vi "Drive_Loop_Drive_Distance.vi"(6 "Distance":dbl, 8 "Absolute Angle? 4":bool, 9 "Angle 3":dbl, 10 "Power 3":dbl, 11 "Drive Loop Cluster":T1) -> ()   [LabVIEW 2016]
doc: "Help file writen by FRC Team 836 - The RoboBees\n\nThis VI commands the robot to drive a certain distance.\n\nThis VI writes the \"Drive Distance\" command, power level #3, Distance to travel, and if it is an absoulute angle to the\nDrive Command RT FIFO in Drive Loop Cluster.\n\nThe RT FIFO has to be initialized using the \"Drive_Loop_Initialize_w_Help\" VI"
uses:
  <userlib>/836-libraries/Drive/Drive_Code/Drive_Code_Support/Drive_Code_Bundle.ctl
  <userlib>/836-libraries/Drive/Drive_Code/Drive_Code_Support/Sensor_Cluster.ctl
  <userlib>/836-libraries/Drive/Drive_Code/Drive_Code_Support/Camera_Cluster.ctl
  <userlib>/836-libraries/Drive/Drive_Code/Drive_Code_Support/Drive_Code_Notifier.ctl
  <userlib>/836-libraries/Drive/Drive_Code/Drive_Code_Support/Drive_Code_Command.ctl
  <userlib>/836-libraries/Drive/Drive_Code/Logging_Data.ctl
  <userlib>/836-libraries/Drive/Drive_Code/Drive_Code_Support/Drive_Code_PID_Bundle.ctl
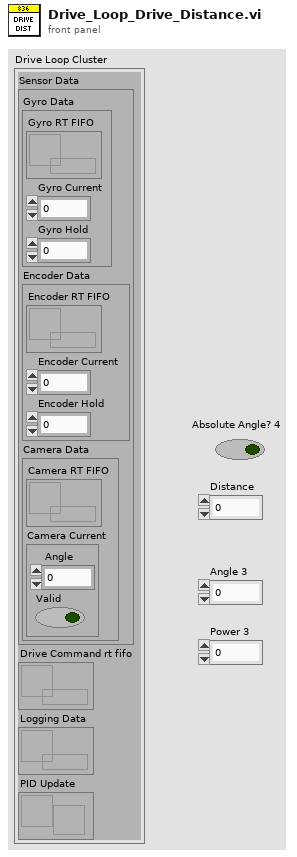
[diagram p1: front panel]
types:
  T1 = typedef "Drive_Code_Bundle.ctl" = cluster{"Sensor Data":T2, "Drive Command rt fifo":refnum<k33>, "Logging Data":refnum<k33>, "PID Update":refnum<notifier>}
  T2 = typedef "Sensor_Cluster.ctl" = cluster{"Gyro Data":cluster{"Gyro RT FIFO":refnum<k33>, "Gyro Current":dbl, "Gyro Hold":dbl}, "Encoder Data":cluster{"Encoder RT FIFO":refnum<k33>, "Encoder Current":dbl, "Encoder Hold":dbl}, "Camera Data":cluster{"Camera RT FIFO":refnum<k33>, "Camera Current":T3}}
  T3 = typedef "Camera_Cluster.ctl" = cluster{" Angle":dbl, "Valid":bool}
  T4 = typedef "Drive_Code_Command.ctl" = enum16{"Do Nothing", "Manual", "Drive Continuous", "Turn", "Drive Distance", "Hold Position", "Hold Yaw", "Follow Camera", "Turn to Camera"}
  T5 = typedef "Drive_Code_Notifier.ctl" = cluster{"Command":T4, "Parameter A":dbl, "Parameter B":dbl, "Parameter C":dbl, "Absolute?":bool}
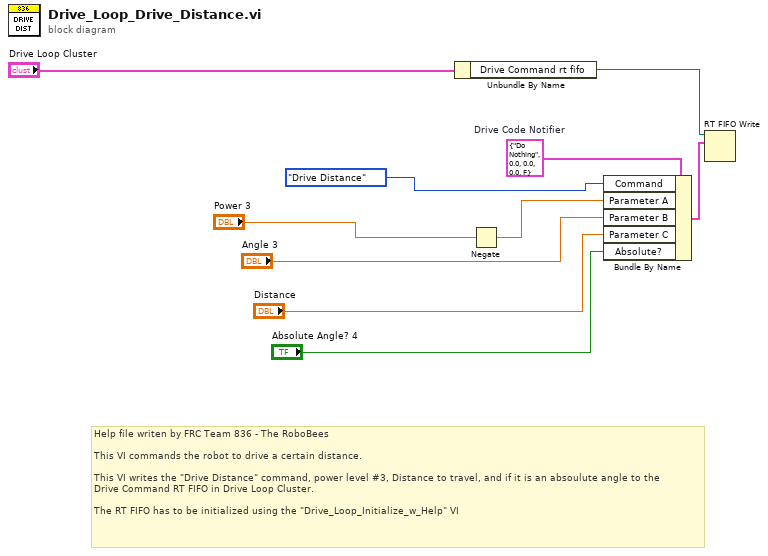
[diagram p0: block diagram]
diagram:
  w1 = T5 {"Command"=enum."Do Nothing", "Parameter A"=0.0, "Parameter B"=0.0, "Parameter C"=0.0, "Absolute?"=FALSE}  # Drive Code Notifier
  # "Help file writen by FRC Team 836 - The RoboBees\n\nThis VI commands the robot to drive a certain distance.\n\nThis VI writes the \"Drive Distance\" command, power level #3, Distance to travel, and if it is an absoulute angle to the\nDrive Command RT FIFO in Drive Loop Cluster.\n\nThe RT FIFO has to be initialized using the \"Drive_Loop_Initialize_w_Help\" VI"
  n1 = Unbundle By Name("Drive Loop Cluster") -> ("Drive Command rt fifo"=w10:refnum<k33>)
  n2 = Negate(x="Power 3") -> (-x=w7:dbl)
  n3 = Bundle By Name(cluster=w1, "Command"=Drive_Code_Command."Drive Distance", "Parameter A"=w7, "Parameter B"="Angle 3", "Parameter C"="Distance", "Absolute?"="Absolute Angle? 4") -> (w9:T5)
  n4 = RT FIFO Write(0:w10, 1:w9) -> ()  [unwired: 3 in, 4 out]
